vi "SOQPSK Demodulator - Channel 1.vi"() -> ()   [LabVIEW 2025]
uses:
  Shared/BER/FPGA/PRBS/PRBS Degree Selection.ctl
  <vilib>/userDefined/High Color/nirio_resource_hc.ctl
  Support/Public/FPGA Refnum.ctl
  <vilib>/DataMovement_sc/v1/host/Buffer/Buffer v1 Host.lvclass
  Shared/Public/Demodulation Control.ctl
  Shared/BER/Host/BER Host.lvclass
  <vilib>/addons/Modulation/Analog/controls/Complex Data Waveform.ctl
  81d51112-337f-4dfa-9d15-b0590b4feb5c.vi
  9fb14cbd-fd79-4d00-90ce-d316e1cdf087.vi
  0a5f839e-e301-4e9c-9aed-57d8c3bb4e49.vi
  <vilib>/FPGAPlugInAG/Dynamic/niLvFpga_Download_Dynamic.vi
  <vilib>/FPGAPlugInAG/Dynamic/niLvFpga_Run_Dynamic.vi
  <vilib>/FPGAPlugInAG/Dynamic/niLvFpga_Close_Dynamic.vi
  <vilib>/rvi/interface/common/niFpgaWaitOnOcc.vi
  <vilib>/Utility/error.llb/Error Cluster From Error Code.vi
  <vilib>/rvi/errors/niLvFpgaAdjustHostInterfaceError.vi
  <vilib>/DLsc/v1/Host/Link Engine/Add Hardware - Single.vi
  <vilib>/DLsc/v1/Host/Link Engine/Get Device Registers - IFW.vi
  <vilib>/DLsc/v1/Host/Protocols/Aurora 64b66b/Extension/Configure RX - Single.vi
  <vilib>/DLsc/v1/Host/Link Engine/Commit Links - Single.vi
  <vilib>/DLsc/v1/Host/Link Engine/Enable Links - Single.vi
  <vilib>/DLsc/v1/Host/Link Engine/Abort Links - Single.vi
  <vilib>/DLsc/v1/Host/Link Engine/Disable Links - Single.vi
  <vilib>/DLsc/v1/Host/Link Engine/Close References - Single.vi
  <vilib>/rvi/interface/nirviMethod/nirviMethod.xnode
  <vilib>/rvi/interface/nirviCloseFPGA/nirviCloseFPGA.xnode
  <vilib>/rvi/interface/nirviReadWriteControl/nirviReadWriteControl.xnode
  <vilib>/rvi/interface/Simulation/niFpgaSimulationCallBeginRW.vi
  <vilib>/FPGAPlugInAG/Dynamic/niLvFpga_ReadFifo_Dynamic.vi
  <vilib>/rvi/errors/niLvFpgaMergeErrorWithErrorCode.vi
  <vilib>/addons/Modulation/niDMT.lvlib
  Support/SOQPSK Host Support.lvlib
  Shared/SOQPSK Modem Shared.lvlib
  <vilib>/addons/Modulation/niAMT.lvlib
  <vilib>/DLsc/v1/Host/Link Engine/DLsc Link Engine v1 Host.lvlib
  <vilib>/DLsc/v1/Host/Protocols/Aurora 64b66b/Extension/Aurora 64b66b Extension.lvlib
  NiFpgaLv.dll
  <vilib>/FPGAPlugInAG/Dynamic/niLvFpga_ConfigureFifo_Dynamic.vi
  <vilib>/FPGAPlugInAG/Dynamic/niLvFpga_StartFifo_Dynamic.vi
  Shared/BER/FPGA/PRBS/PRBS.lvlib
panel:
  out "Actual Symbol Rate (Hz)":dbl caption="actual symbol rate" format="%#_6p"
  out "Bitfile Redownloaded":bool
  in  "Coprocessor Device Name":T1
  in  "Signal Parameters":T3={"Symbol Rate (Hz)"=18000000.0, "Pulse Parameters"={"Payload Length"=500, "Preamble Symbol"=449838109, "PN Order"=0}} {"Pulse Parameters"."PN Order" items=["7", "9", "10", "11", "15", "17", "18", "20", "21", "22", "23", "25"]; "Pulse Parameters"."Preamble Symbol" format="%.0x"; "Symbol Rate (Hz)" format="%#_6p"}
  in  "Coprocessor Bitfile Path":path
  out "Constellation":T4(graph) caption="IQ Constellation"
  out "BER FPGA":dbl caption="Bit Error Rate" format="%.6f%%"
  out "IQ Rate (S/s)":dbl format="%#_6p"
  in  "Reset BER":bool
  out "Samples per Symbol":i32
  in  "stop":bool
  out "Status":string
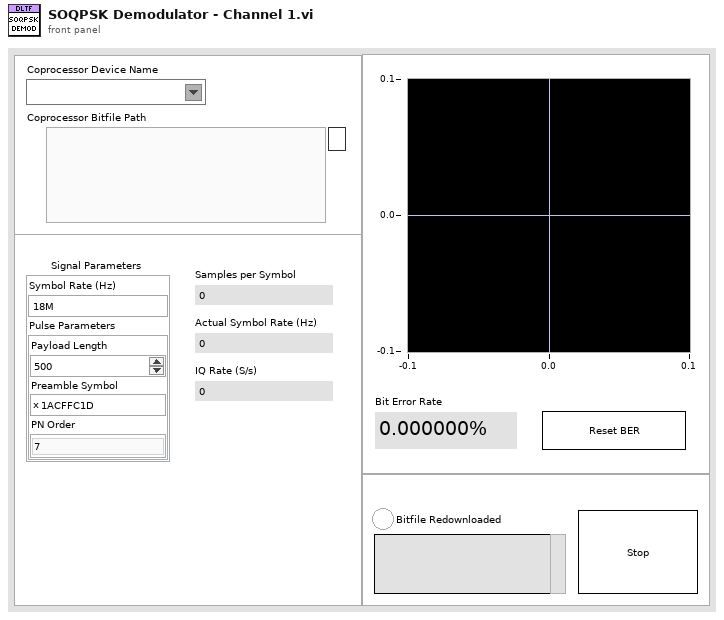
[diagram p1: front panel]
types:
  T1 = typedef "nirio_resource_hc.ctl" = tag
  T2 = typedef "Modems Shared.lvlib/PRBS.lvlib/PRBS Degree Selection.ctl" = u16
  T3 = cluster{"Symbol Rate (Hz)":dbl, "Pulse Parameters":cluster{"Payload Length":u16, "Preamble Symbol":i32, "PN Order":T2}}
  T4 = cluster{"constellation":dbl[], "oversampled data":dbl[]}[]
  T5 = typedef "SOQPSK Host Support.lvlib/FPGA Refnum.ctl" = refnum<k20>
  T6 = typedef "DLsc Link Engine v1 Host.lvlib/DLsc Session.lvclass/Session Handle.ctl" = refnum<data-value>
  T7 = typedef "DLsc Link Engine v1 Host.lvlib/DLsc Session.lvclass/Device Address Information.ctl" = cluster{"device name":string, "bitfile path":path}
  T8 = typedef "IFW Session v1 Host.lvlib/IFW Session.ctl" = cluster{"refnum":refnum<k20>, "subsystem map":refnum<class "niInstr Subsystem Map v1 Host.lvclass">, "register bus":refnum<class "niInstr FIFO Register Bus v1 Host.lvclass">, "IFW subsystems":T9}
  T9 = typedef "IFW Session v1 Host.lvlib/IFW Subsystems.ctl" = cluster{"IFW address space collection":T10}[]
  T10 = typedef "IFW Session v1 Host.lvlib/IFW Address Space Collection.ctl" = T11[]
  T11 = typedef "IFW Session v1 Host.lvlib/IFW Address Space.ctl" = cluster{"name":string, "IFW address space information":T12, "class path":path}
  T12 = typedef "IFW Session v1 Host.lvlib/IFW Address Space Information.ctl" = cluster{"UID":u16, "instance":u8}
  T13 = typedef "SOQPSK Modem Shared.lvlib/Demodulation Control.ctl" = i16
  T14 = cluster{"[0]":fxp<+/-,16,1>, "[1]":fxp<+/-,16,1>, "[2]":fxp<+/-,16,1>, "[3]":fxp<+/-,16,1>, "[4]":fxp<+/-,16,1>, "[5]":fxp<+/-,16,1>, "[6]":fxp<+/-,16,1>, "[7]":fxp<+/-,16,1>, "[8]":fxp<+/-,16,1>, "[9]":fxp<+/-,16,1>, "[10]":fxp<+/-,16,1>, "[11]":fxp<+/-,16,1>, "[12]":fxp<+/-,16,1>, "[13]":fxp<+/-,16,1>, "[14]":fxp<+/-,16,1>, "[15]":fxp<+/-,16,1>, "[16]":fxp<+/-,16,1>}
  T15 = typedef "niAMT.lvlib/Complex Data Waveform.ctl" = cluster{"t0":dbl, "dt":dbl, "Y":cdb[]}
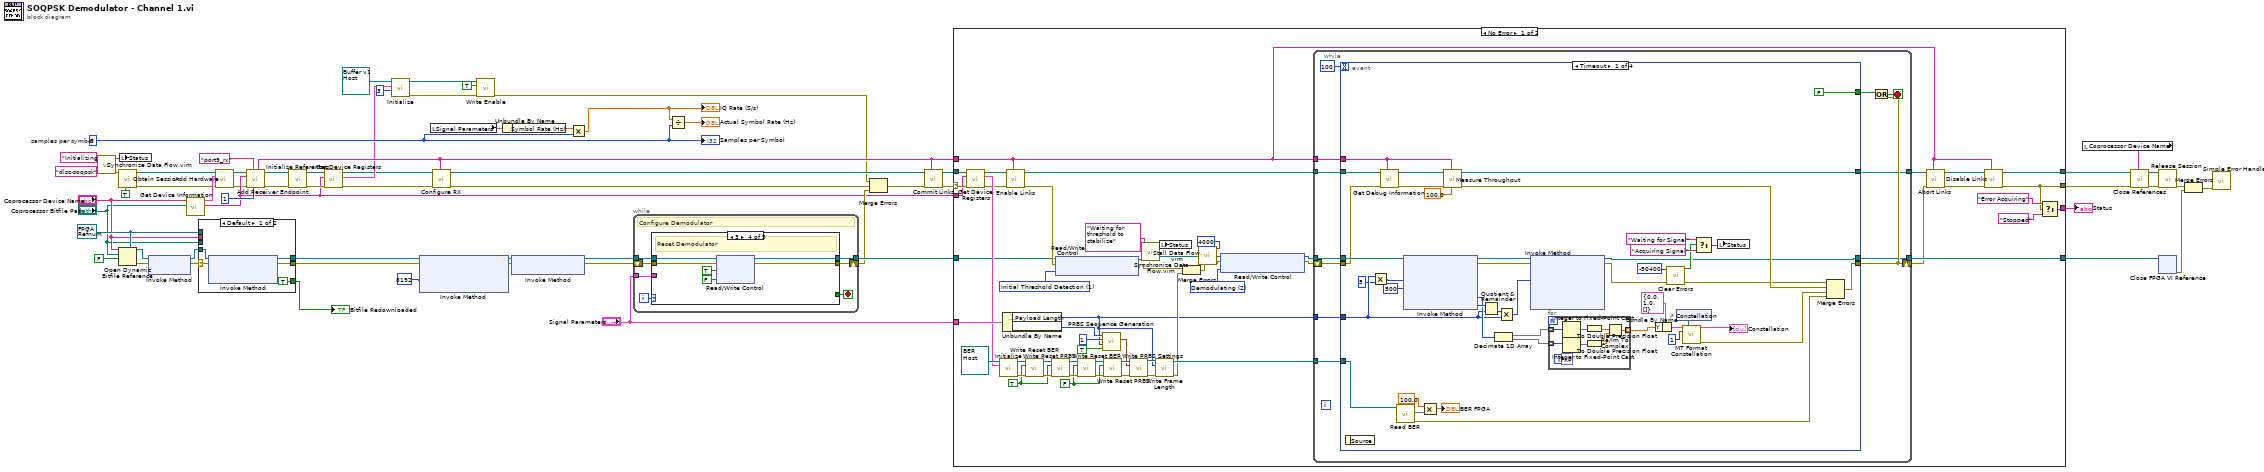
[diagram p0: block diagram]
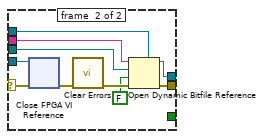
[diagram p2: hidden frame]
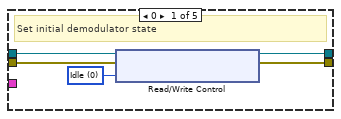
[diagram p3: hidden frame]
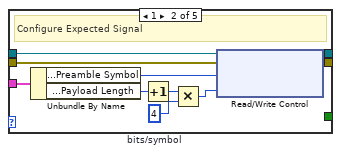
[diagram p4: hidden frame]
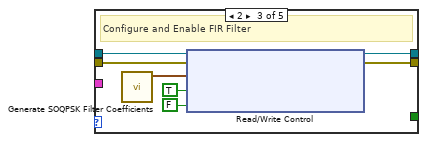
[diagram p5: hidden frame]
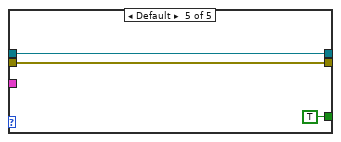
[diagram p6: hidden frame]
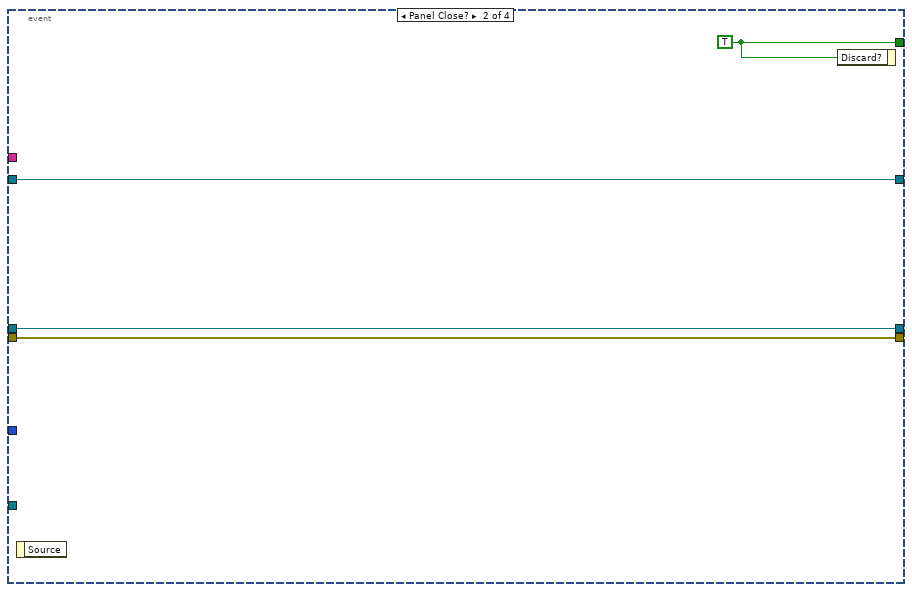
[diagram p7: hidden frame]
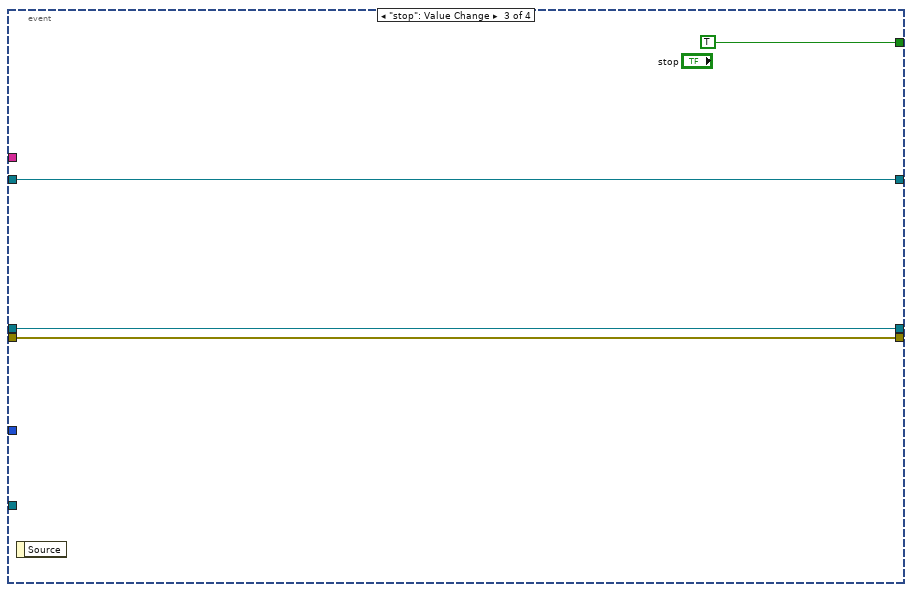
[diagram p8: hidden frame]
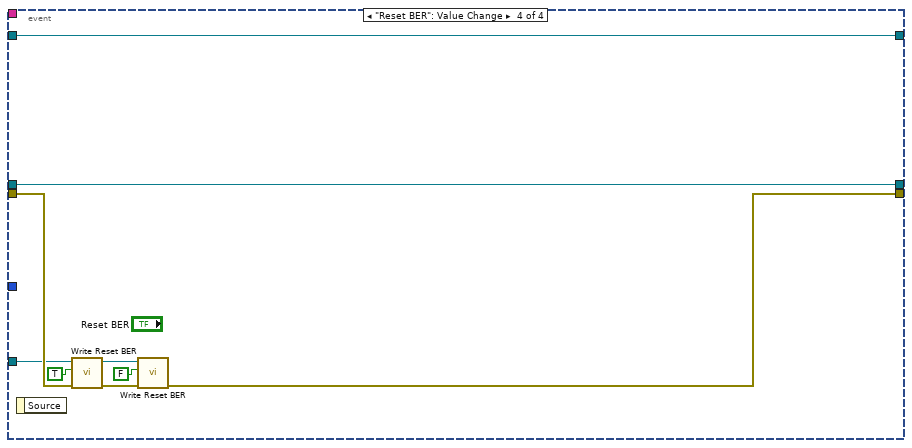
[diagram p9: hidden frame]
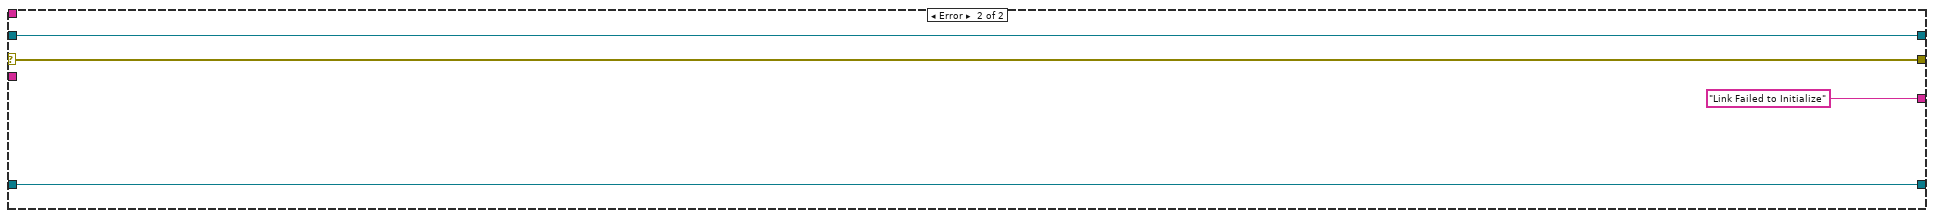
[diagram p10: hidden frame]
diagram:
  w51 = T5 refnum ("datalink soqpsk fpga refnum")
  w37 = 8  # samples per symbol
  n1 = call "Synchronize Data Flow.vim"("input 4"="dlsc-soqpsk" ("session name"), "input 1"="Initializing") -> ("output 4"=w40:string, "output 1"=w39:string)  [unwired: 2 in, 2 out]
  n2 = call <vilib>:"Obtain Session.vi"("use remote engine (f)"=TRUE, "session name (\"\":default)"=w40) -> ("error out"=w9:errorcluster, "session out"=w10:T6)  [unwired: 6 in, 2 out]
  n3 = Open Dynamic Bitfile Reference(0:"Coprocessor Device Name", 1:"Coprocessor Bitfile Path", 2:FALSE ("Run When Loaded"), 4:w51) -> (5:w50:T5, 8:w49:errorcluster)  [unwired: 1 in]
  n4 = local write "Status"(w39) -> ()
  n5 = xnode "Invoke Method"("FPGA VI Reference In"=w50, "error in"=w49) -> ("FPGA VI Reference Out"=w53:T5, "error out"=w52:errorcluster)
  n6 = call <vilib>:"Get Device Information.vi"("bitfile path"="Coprocessor Bitfile Path", "device name"="Coprocessor Device Name") -> ("device name out"=w16:string, "device address information"=w43:T7)  [unwired: 7 in, 1 out]
  n7 = case shown="Default" w52 {
    selector: w52 -> [w69 w81]
    tunnel: [w71 w74] -> w2
    tunnel: [w70 w77] -> w1
    tunnel: w53 -> [w68 w79]
    tunnel: w51 -> [_ w75]
    tunnel: "Coprocessor Device Name" -> [_ w73]
    tunnel: "Coprocessor Bitfile Path" -> [_ w72]
    tunnel: [TRUE _] -> w48
    frame #0 {
      n8 = xnode "Invoke Method"("FPGA VI Reference In"=w68, "error in"=w69) -> ("FPGA VI Reference Out"=w71:T5, "error out"=w70:errorcluster)  [unwired: 1 in]
    }
    frame #1 {
      n9 = xnode "Close FPGA VI Reference"("FPGA VI Reference In"=w79, "error in"=w81) -> ("error out"=w80:errorcluster)
      n10 = call <vilib>:"Clear Errors.vi"("error in (no error)"=w80) -> ("error out"=w78:errorcluster)  [unwired: 5 in, 1 out]
      n11 = Open Dynamic Bitfile Reference(0:w73, 1:w72, 2:FALSE ("Run When Loaded"), 3:w78, 4:w75) -> (5:w74:T5, 8:w77:errorcluster)
    }
  }
  "Bitfile Redownloaded" <- w48
  n12 = call-poly <vilib>:"Add Hardware.vi"("error in"=w9, "device"=w43, "session in"=w10) -> ("error out"=w8:errorcluster, "session out"=w7:T6)  [unwired: 7 in]
  n13 = call <vilib>:"Add Receiver Endpoint.vi"("receiver instance (0)"=u8 1, "link name"="port9_rx", "error in"=w8, "receiver device name"=w16, "session in"=w7) -> ("error out"=w5:errorcluster, "session out"=w6:T6, "link name out"=w23:string)  [unwired: 2 in, 2 out]
  n14 = call <vilib>:"Initialize References.vi"("error in"=w5, "session in"=w6) -> ("error out"=w18:errorcluster, "session out"=w17:T6)  [unwired: 8 in]
  n15 = call-poly <vilib>:"Get Device Registers.vi"("error in"=w18, "hardware name"=w16, "session in"=w17) -> ("error out"=w3:errorcluster, "ifw session"=w15:T8, "session out"=w4:T6)  [unwired: 6 in]
  n16 = call-dynamic "Initialize.vi"("instance(0)"=u8 3, "session"=w15, "ifw address space collection host in"=refnum<class "Buffer v1 Host.lvclass"> refnum ("Buffer v1 Host.lvclass")) -> ("error out"=w20:errorcluster, "ifw address space collection host out"=w21:refnum<class "Buffer v1 Host.lvclass">)  [unwired: 6 in, 1 out]
  n17 = xnode "Invoke Method"("FPGA VI Reference In"=w2, "error in"=w1, "Requested Depth"=u32 8192) -> ("FPGA VI Reference Out"=w65:T5, "error out"=w66:errorcluster)  [unwired: 1 out]
  n18 = local read "Signal Parameters"() -> (w38:T3)
  n19 = call-poly <vilib>:"Configure RX.vi"("link name (\"\":default)"=w23, "error in"=w3, "session in"=w4) -> ("error out"=w24:errorcluster, "session out"=w14:T6)  [unwired: 7 in]
  n20 = call <vilib>:"Write Enable.vi"("error in"=w20, "enable (f)"=TRUE, "buffer v1 host in"=w21) -> ("error out"=w12:errorcluster)  [unwired: 7 in, 1 out]
  n21 = Unbundle By Name(w38) -> ("Symbol Rate (Hz)"=w63:dbl)
  n22 = xnode "Invoke Method"("FPGA VI Reference In"=w65, "error in"=w66) -> ("FPGA VI Reference Out"=w57:T5, "error out"=w56:errorcluster)
  n23 = Multiply(x=w63, y=w37) -> (x*y=w29:dbl)
  "IQ Rate (S/s)" <- w29
  n24 = while {
    tunnel: [w87] -> w55
    shift-right: [w86] -> w44
    shift-left: w56 -> [w84]
    tunnel: w57 -> [w85]
    tunnel: "Signal Parameters" -> [w83]
    i -> [w88]
    stop <- w82 stop-if-true
    # "Configure Demodulator"
    n25 = case shown="3" w88 {
      tunnel: [w92 w100 w109 w115 w119] -> w87
      tunnel: [w91 w99 w108 w114 w118] -> w86
      tunnel: w85 -> [w90 w103 w110 w116 w119]
      tunnel: w84 -> [w89 w94 w105 w112 w118]
      tunnel: w83 -> [_ w102 _ _ _]
      tunnel: [_ _ _ _ TRUE] -> w82
      frame 0 {
        w93 = T13 0 items=["Idle", "Initial Threshold Detection", "Demodulating"] ("demodulation control")
        # "Set initial demodulator state"
        n26 = xnode "Read/Write Control"("FPGA VI Reference In"=w90, "error in"=w89, "demodulation control.1"=w93) -> ("FPGA VI Reference Out"=w92:T5, "error out"=w91:errorcluster)
      }
      frame 1 {
        w95 = 4  # bits/symbol
        # "Configure Expected Signal"
        n27 = Unbundle By Name(w102) -> ("Pulse Parameters.Preamble Symbol"=w101:i32, "Pulse Parameters.Payload Length"=w98:u16)
        n28 = Increment(x=w98) -> (x+1=w96:u16)
        n29 = Multiply(x=w96, y=w95) -> (x*y=w97:i32)
        n30 = xnode "Read/Write Control"("FPGA VI Reference In"=w103, "error in"=w94, "preamble.1"=w101, "payload length.1"=w97) -> ("FPGA VI Reference Out"=w100:T5, "error out"=w99:errorcluster)
      }
      frame 2 {
        # "Configure and Enable FIR Filter"
        n31 = call "Generate SOQPSK Filter Coefficients.vi"() -> ("symmetric filter coefficients"=w107:T14)  [unwired: 7 in, 4 out]
        n32 = xnode "Read/Write Control"("FPGA VI Reference In"=w110, "error in"=w105, "symmetric filter coefficients .1"=w107, "enable match filter.1"=TRUE ("enable match filter"), "enable match filter.1"=FALSE ("enable match filter.0")) -> ("FPGA VI Reference Out"=w109:T5, "error out"=w108:errorcluster)
      }
      frame 3 {
        # "Reset Demodulator"
        n33 = xnode "Read/Write Control"("FPGA VI Reference In"=w116, "error in"=w112, "reset rx.1"=TRUE ("reset demodulator"), "reset rx.1"=FALSE ("enable match filter")) -> ("FPGA VI Reference Out"=w115:T5, "error out"=w114:errorcluster)
      }
      frame Default {
      }
    }
  }
  n34 = Divide(x=w29, y=w37) -> (x/y=→"Actual Symbol Rate (Hz)":dbl)
  n35 = Merge Errors(w12, w24, w44) -> (w13:errorcluster)
  n36 = call-poly <vilib>:"Commit Links.vi"("link name (\"\":all)"=w23, "error in"=w13, "session in"=w14) -> ("error out"=w58:errorcluster, "session out"=w59:T6)  [unwired: 7 in]
  n37 = case shown="No Error" w58 {
    selector: w58 -> [w168 w257]
    tunnel: w59 -> [w169 w258]
    tunnel: [w122 w258] -> w27
    tunnel: [w121 w257] -> w26
    tunnel: w55 -> [w135 w256]
    tunnel: [w174 w256] -> w62
    tunnel: w23 -> [w120 _]
    tunnel: "Signal Parameters" -> [w170 _]
    tunnel: w16 -> [w167 _]
    tunnel: [w145 "Link Failed to Initialize" ("t")] -> w35
    frame No Error {
      w131 = T13 2 items=["Idle", "Initial Threshold Detection", "Demodulating"] ("demodulation control")
      w137 = T13 1 items=["Idle", "Initial Threshold Detection", "Demodulating"] ("demodulation control")
      w154 = FALSE ("reset")
      w153 = TRUE ("reset")
      n38 = call-poly <vilib>:"Get Device Registers.vi"("error in"=w168, "hardware name"=w167, "session in"=w169) -> ("error out"=w142:errorcluster, "ifw session"=w144:T8, "session out"=w143:T6)  [unwired: 6 in]
      n39 = call-dynamic "Initialize.vi"("session"=w144, "ifw address space collection host in"=refnum<class "BER Host.lvclass"> refnum ("BER")) -> ("error out"=w159:errorcluster, "ifw address space collection host out"=w160:refnum<class "BER Host.lvclass">)  [unwired: 7 in, 1 out]
      n40 = Unbundle By Name(w170) -> ("Pulse Parameters.Payload Length"=w148:u16, "Pulse Parameters.PN Order"=w172:T2)
      n41 = call-poly <vilib>:"Enable Links.vi"("link name (\"\":all)"=w120, "error in"=w142, "session in"=w143) -> ("error out"=w136:errorcluster, "session out"=w141:T6)  [unwired: 7 in]
      n42 = call "Write Reset BER.vi"("error in"=w159, "reset"=w153, "BER"=w160) -> ("error out"=w162:errorcluster, "BER out"=w161:refnum<class "BER Host.lvclass">)  [unwired: 7 in]
      n43 = call "Write Reset PRBS.vi"("error in"=w162, "reset"=w153, "BER"=w161) -> ("error out"=w163:errorcluster, "BER out"=w164:refnum<class "BER Host.lvclass">)  [unwired: 7 in]
      n44 = xnode "Read/Write Control"("FPGA VI Reference In"=w135, "error in"=w136, "demodulation control.1"=w137) -> ("FPGA VI Reference Out"=w140:T5, "error out"=w134:errorcluster)
      n45 = call "Write Reset BER.vi"("error in"=w163, "reset"=w154, "BER"=w164) -> ("error out"=w166:errorcluster, "BER out"=w165:refnum<class "BER Host.lvclass">)  [unwired: 7 in]
      n46 = call "PRBS Sequence Generation.vi"("backward"=TRUE, "total bits"=w148, "seed"=u32 1, "PRBS degree"=w172) -> ("PRBS setting"=w149:cluster{"degree":u8, "tap":u8, "seed":u32})  [unwired: 6 in, 1 out]
      n47 = call "Write Reset PRBS.vi"("error in"=w166, "reset"=w154, "BER"=w165) -> ("error out"=w156:errorcluster, "BER out"=w155:refnum<class "BER Host.lvclass">)  [unwired: 7 in]
      n48 = call "Write PRBS Settings.vi"("error in"=w156, "PRBS Settings"=w149, "BER"=w155) -> ("error out"=w157:errorcluster, "BER out"=w158:refnum<class "BER Host.lvclass">)  [unwired: 7 in]
      n49 = call "Synchronize Data Flow.vim"("input 4"=w140, "input 1"="Waiting for threshold to stabilize" ("Status")) -> ("output 4"=w130:T5, "output 1"=w139:string)  [unwired: 2 in, 2 out]
      n50 = call "Write Frame Length.vi"("error in"=w157, "frame length"=w148, "BER"=w158) -> ("error out"=w150:errorcluster, "BER out"=w151:refnum<class "BER Host.lvclass">)  [unwired: 7 in]
      n51 = local write "Status"(w139) -> ()
      n52 = Merge Errors(w134, w150) -> (w127:errorcluster)
      n53 = call "Stall Data Flow.vim"("value in"=w130, "milliseconds to wait"=u32 4000) -> ("value out"=w133:T5)  [unwired: 1 out]
      n54 = xnode "Read/Write Control"("FPGA VI Reference In"=w133, "error in"=w127, "demodulation control.1"=w131) -> ("FPGA VI Reference Out"=w129:T5, "error out"=w128:errorcluster)
      n55 = while {
        shift-right: [w184] -> w123
        shift-left: w128 -> [w182]
        tunnel: w148 -> [w186]
        tunnel: w129 -> [w183]
        tunnel: w141 -> [w179]
        tunnel: [w178] -> w124
        tunnel: [w177] -> w174
        tunnel: w120 -> [w176]
        tunnel: w151 -> [w175]
        stop <- w185 stop-if-true
        n56 = event shown="[0] Timeout" {
          selector: _ -> [_ _ _ _]
          dyn-events: _ -> [_ _ _ _]
          timeout: 100 -> [_ _ _ _]
          tunnel: w186 -> [w189 _ _ _]
          tunnel: [w229 w241 w244 w249] -> w184
          tunnel: w183 -> [w223 w240 w242 w248]
          tunnel: w182 -> [w213 w241 w244 w254]
          tunnel: [FALSE ("stop") w238 TRUE ("stop") _] -> w181
          tunnel: w179 -> [w218 w239 w243 w247]
          tunnel: [w216 w239 w243 w247] -> w178
          tunnel: [w197 w240 w242 w248] -> w177
          tunnel: w176 -> [w217 _ _ _]
          tunnel: w175 -> [w222 _ _ w246]
          event Timeout {
            n57 = event-data() -> ()  [unwired: 1 in, 1 out]
            n58 = Multiply(x=w189, y=u16 5) -> (x*y=w190:u16)
            n59 = call <vilib>:"Get Debug Information.vi"("link name"=w217, "error in"=w213, "session in"=w218) -> ("error out"=w220:errorcluster, "session out"=w219:T6)  [unwired: 5 in, 2 out]
            n60 = call "Read BER.vi"("BER"=w222) -> ("error out"=w224:errorcluster, "BER"=w226:fxp<+,32,0>)  [unwired: 8 in, 1 out]
            n61 = xnode "Invoke Method"("FPGA VI Reference In"=w223, "Number of Elements"=w190, "Timeout (ms)"=500) -> ("FPGA VI Reference Out"=w210:T5, "error out"=w203:errorcluster, "Data"=w193:i32[], "Elements Remaining"=w200:u32)  [unwired: 1 in]
            n62 = Multiply(x=100.0, y=w226) -> (x*y=→"BER FPGA":dbl)
            n63 = call <vilib>:"Measure Throughput.vi"("measurement interval (500ms)"=100.0 ("thruput meas time (ms)"), "link name"=w217, "error in"=w220, "session in"=w219) -> ("error out"=w215:errorcluster, "session out"=w216:T6)  [unwired: 4 in, 2 out]
            n64 = Quotient & Remainder(x=w200, y=w189) -> (floor(x/y)=w209:u32)  [unwired: 1 out]
            n65 = Decimate 1D Array(w193) -> (w195:i32[], w194:i32[])
            n66 = Multiply(x=w209, y=w189) -> (x*y=w196:u32)
            n67 = xnode "Invoke Method"("FPGA VI Reference In"=w210, "error in"=w203, "Number of Elements"=w196) -> ("FPGA VI Reference Out"=w197:T5, "error out"=w199:errorcluster)  [unwired: 1 in, 2 out]
            n68 = for {
              tunnel: [w237] -> w192 mode=indexing
              tunnel: w195 -> [w236] mode=indexing
              tunnel: w194 -> [w235] mode=indexing
              w230 = fxp<+/-,32,4> 0.0
              n69 = Integer to Fixed-Point Cast(fixed-point type=w230, integer=w236) -> (fixed-point=w234:fxp<+/-,32,4>)
              n70 = Integer to Fixed-Point Cast(fixed-point type=w230, integer=w235) -> (fixed-point=w232:fxp<+/-,32,4>)
              n71 = To Double Precision Float(number=w234) -> (double precision float=w233:dbl)
              n72 = To Double Precision Float(number=w232) -> (double precision float=w231:dbl)
              n73 = Re/Im To Complex(1:w231, 2:w233) -> (0:w237:cdb)
            }
            n74 = Bundle By Name(cluster=T15 {"t0"=0.0, "dt"=1.0, "Y"=[]} ("waveform"), "Y"=w192) -> (w202:T15)
            n75 = call <vilib>:"Clear Errors.vi"("error in (no error)"=w199, "specific error code to clear (0: all)"=-50400) -> ("error out"=w198:errorcluster, "specific error cleared?"=w205:bool)  [unwired: 4 in]
            n76 = control-ref of="Constellation"() -> (w212:refnum<vi>)
            n77 = call <vilib>:"MT Format Constellation.vi"("waveform"=w202, "constellation reference"=w212, "samples per symbol"=1) -> ("constellation graph"=→"Constellation":T4, "error out"=w228:errorcluster)  [unwired: 2 in, 9 out]
            n78 = Select(t="Waiting for Signal", s=w205, f="Acquiring Signal") -> (s? t:f=w204:string)
            n79 = local write "Status"(w204) -> ()
            n80 = Merge Errors(w198, w215, w228, w224) -> (w229:errorcluster)
          }
          event Panel Close? {
            w238 = TRUE ("stop")
            n81 = event-data() -> ()  [unwired: 1 in, 1 out]
            n82 = event-data("Discard?"=w238) -> ()  [unwired: 1 in, 1 out]
          }
          event "stop": Value Change {
            n83 = event-data() -> ()  [unwired: 1 in, 1 out]
          }
          event "Reset BER": Value Change {
            n84 = event-data() -> ()  [unwired: 1 in, 1 out]
            n85 = call "Write Reset BER.vi"("error in"=w254, "reset"=TRUE, "BER"=w246) -> ("error out"=w252:errorcluster, "BER out"=w251:refnum<class "BER Host.lvclass">)  [unwired: 7 in]
            n86 = call "Write Reset BER.vi"("error in"=w252, "reset"=FALSE, "BER"=w251) -> ("error out"=w249:errorcluster)  [unwired: 7 in, 1 out]
          }
        }
        n87 = Or(x=w181, y=w184) -> (x .or. y?=w185:bool)
      }
      n88 = call-poly <vilib>:"Abort Links.vi"("link name (\"\":all)"=w120, "error in"=w123, "session in"=w124) -> ("error out"=w126:errorcluster, "session out"=w125:T6)  [unwired: 7 in]
      n89 = call-poly <vilib>:"Disable Links.vi"("link name (\"\":all)"=w120, "error in"=w126, "session in"=w125) -> ("error out"=w121:errorcluster, "session out"=w122:T6)  [unwired: 7 in]
      n90 = Select(t="Error Acquiring", s=w121, f="Stopped") -> (s? t:f=w145:string)
    }
    frame Error {
    }
  }
  "Status" <- w35
  n91 = local read "Coprocessor Device Name"() -> (w32:T1)
  n92 = call-poly <vilib>:"Close References.vi"("device name"=w32, "error in"=w26, "session in"=w27) -> ("error out"=w33:errorcluster, "session out"=w34:T6)  [unwired: 7 in]
  n93 = call <vilib>:"Release Session.vi"("error in"=w33, "session in"=w34) -> ("error out"=w31:errorcluster)  [unwired: 8 in, 1 out]
  n94 = xnode "Close FPGA VI Reference"("FPGA VI Reference In"=w62) -> ("error out"=w60:errorcluster)  [unwired: 1 in]
  n95 = Merge Errors(w31, w60) -> (w61:errorcluster)
  n96 = call <vilib>:"Simple Error Handler.vi"("error in (no error)"=w61) -> ()  [unwired: 4 in, 5 out]
  "Samples per Symbol" <- w37
